vi "IkiOffset.vi"() -> ()   [LabVIEW 2009]
panel:
  in  "Y offset":dbl=5.0
  in  "Iki Name":string="ohanaiki2"
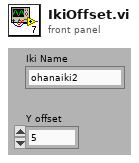
[diagram p1: front panel]
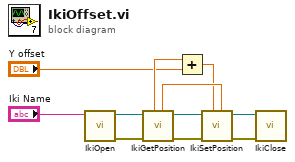
[diagram p0: block diagram]
diagram:
  n1 = call "IkiOpen.vi"("Iki Name"="Iki Name") -> ("error out"=w10:errorcluster, "connection ID"=w9:refnum<k5>)  [unwired: 7 in]
  n2 = call "IkiGetPosition.vi"("error in (no error)"=w10, "connection ID"=w9) -> ("error out"=w7:errorcluster, "connection ID out"=w8:refnum<k5>, "Y"=w3:dbl, "X"=w4:dbl)  [unwired: 4 in]
  n3 = Add(x=w4, y="Y offset") -> (x+y=w2:dbl)
  n4 = call "IkiSetPosition.vi"("Y"=w3, "X"=w2, "error in (no error)"=w7, "connection ID"=w8) -> ("error out"=w6:errorcluster, "connection ID out"=w5:refnum<k5>)  [unwired: 4 in]
  n5 = call "IkiClose.vi"("error in (no error)"=w6, "connection ID"=w5) -> ()  [unwired: 7 in, 1 out]
